vi "write_attributes.vi"(8 "error in (no error)":errorcluster, 10 "attributes":T1, 11 "MiniBatchDictionaryLearning in":refnum<class "MiniBatchDictionaryLearning.lvclass">) -> (0 "error out":errorcluster, 3 "MiniBatchDictionaryLearning out":refnum<class "MiniBatchDictionaryLearning.lvclass">)   [LabVIEW 2020, in "MiniBatchDictionaryLearning.lvclass"]
uses:
  MiniBatchDictionaryLearning.lvclass
  Controls/mini_batch_dictionary_learning_attributes.ctl
  MiniBatchDictionaryLearning.lvclass/MiniBatchDictionaryLearning.ctl
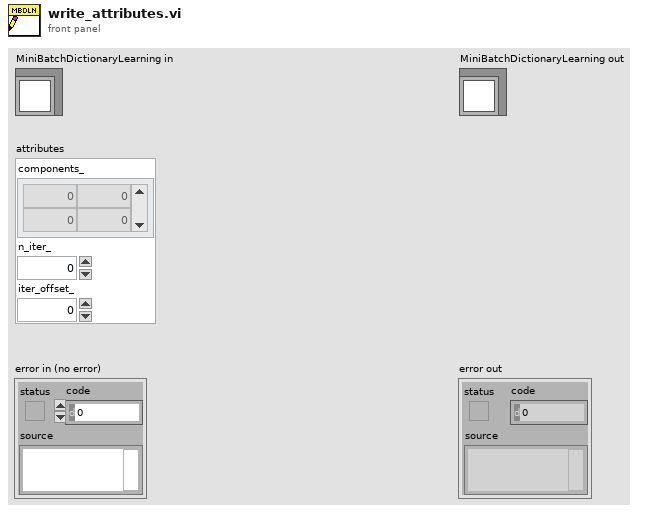
[diagram p1: front panel]
types:
  T1 = typedef "mini_batch_dictionary_learning_attributes.ctl" = cluster{"components_":dbl[][], "n_iter_":dbl, "iter_offset_":dbl}
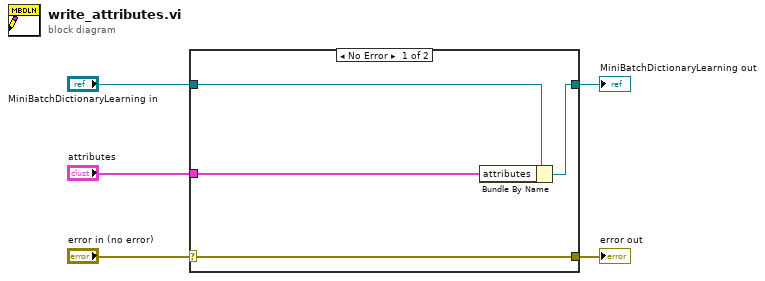
[diagram p0: block diagram]
diagram:
  n1 = case shown="No Error" "error in (no error)" {
    selector: "error in (no error)" -> [w9 w10]
    tunnel: [w9 w10] -> w4
    tunnel: [w7 w11] -> w2
    tunnel: "MiniBatchDictionaryLearning in" -> [w8 w11]
    tunnel: "attributes" -> [w6 _]
    frame No Error {
      n2 = Bundle By Name(cluster=w8, "attributes"=w6) -> (w7:refnum<class "MiniBatchDictionaryLearning.lvclass">)
    }
    frame Error {
    }
  }
  "error out" <- w4
  "MiniBatchDictionaryLearning out" <- w2
